vi "connect.vi"(0 "reference":refnum<class "AbstractEdge.lvclass">, 1 "startNode":refnum<class "AbstractNode.lvclass">, 2 "endNode":refnum<class "AbstractNode.lvclass">, 5 "error in (no error)":errorcluster) -> (14 "reference out":refnum<class "AbstractEdge.lvclass">, 19 "error out":errorcluster)   [LabVIEW 2014, in "AbstractEdge.lvclass"]
doc: "public void connect(Node s, Node e)"
uses:
  <resource>/Framework/Providers/Open_GDS/UML/AbstractEdge_class/AbstractEdge.lvclass
  <resource>/Framework/Providers/Open_GDS/UML/AbstractNode_class/AbstractNode.lvclass
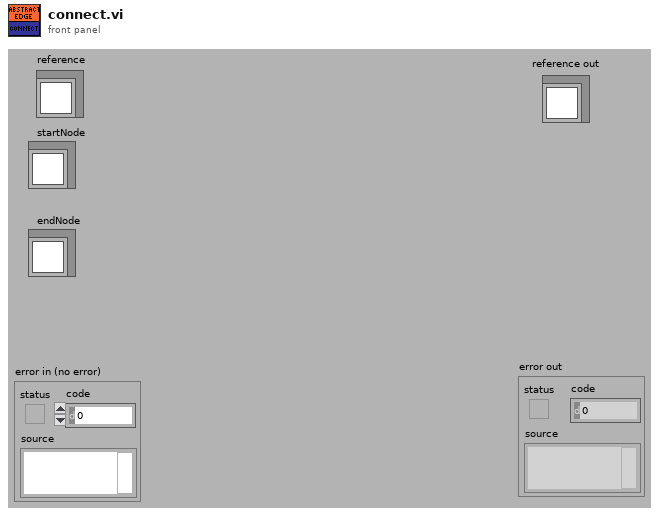
[diagram p1: front panel]
types:
  T1 = typedef "AbstractEdge.lvclass/ObjectAttributes.ctl" = cluster{"start":refnum<class "AbstractNode.lvclass">, "end":refnum<class "AbstractNode.lvclass">}
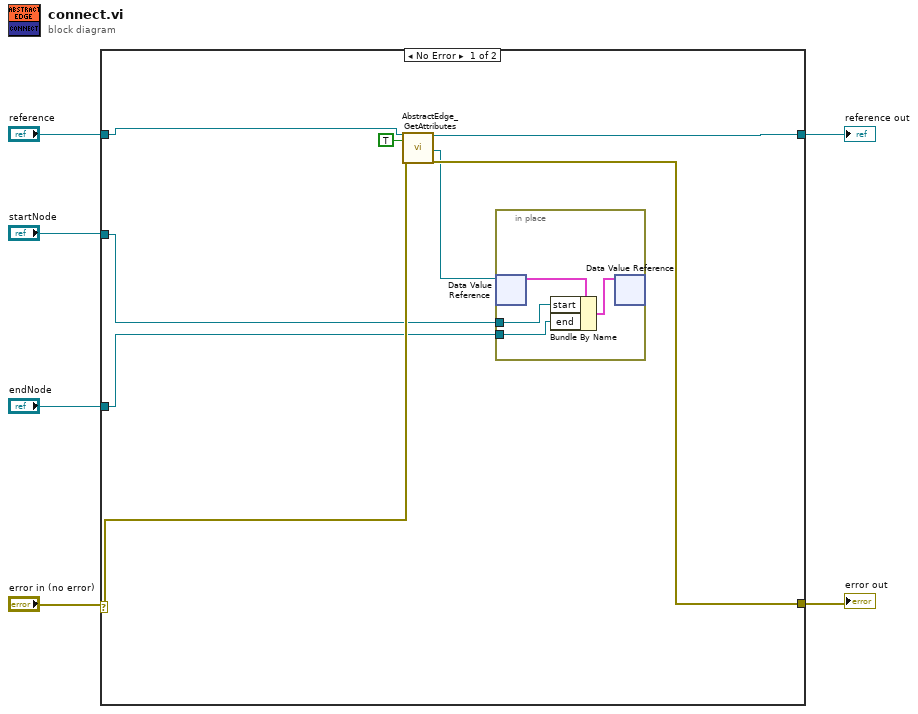
[diagram p0: block diagram]
diagram:
  n1 = case shown="No Error" "error in (no error)" {
    selector: "error in (no error)" -> [w11 w19]
    tunnel: "reference" -> [w14 w20]
    tunnel: [w13 w19] -> w5
    tunnel: [w12 w20] -> w4
    tunnel: "startNode" -> [w8 _]
    tunnel: "endNode" -> [w7 _]
    frame No Error {
      n2 = call <resource>:"AbstractEdge_GetAttributes.vi"("reference in"=w14, "OnlyGetDvrReference(False)"=TRUE, "error in (no error)"=w11) -> ("reference out"=w12:refnum<class "AbstractEdge.lvclass">, "DataRef"=w9:refnum<data-value>, "error out"=w13:errorcluster)  [unwired: 13 in, 1 out]
      n3 = in-place {
        in-place-border: w8 -> [w17]
        in-place-border: w7 -> [w16]
        n4 = in-place-dvr #1(w9) -> (w18:T1)  [unwired: 1 out]
        n5 = Bundle By Name(cluster=w18, "start"=w17, "end"=w16) -> (w15:T1)
        n6 = in-place-dvr #1(w15) -> ()  [unwired: 2 out]
      }
    }
    frame Error {
    }
  }
  "reference out" <- w4
  "error out" <- w5
